vi "Destroy.vi"(8 "error in (no error)":errorcluster, 11 "Array In":refnum<class "Array.lvclass">) -> (0 "error out":errorcluster, 7 "MapImp out":refnum<class "Array.lvclass">)   [LabVIEW 2013, in "LapDog.Collections.v_.Maps.Implementations.lvlib" / "Array.lvclass"]
uses:
  Array.lvclass
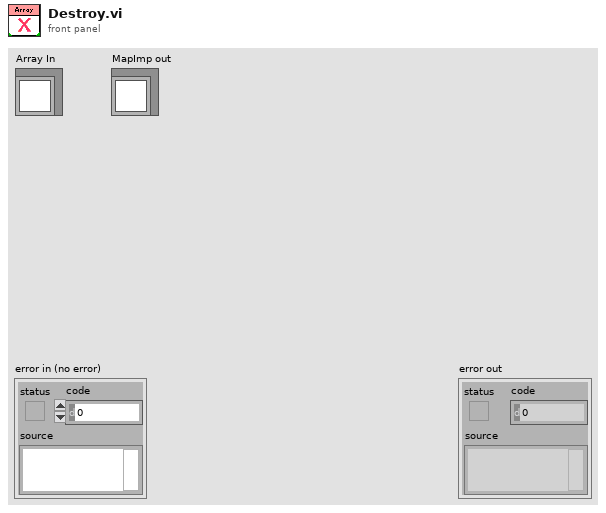
[diagram p1: front panel]
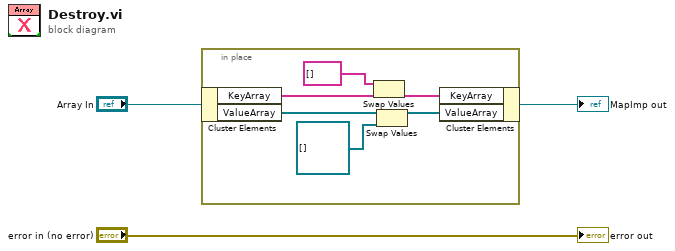
[diagram p0: block diagram]
diagram:
  n1 = in-place {
    n2 = in-place-cluster #1("Array In") -> ("KeyArray"=w7:string[], "ValueArray"=w5:refnum<class>[])
    n3 = Swap Values(12:string[] [] ("KeyArray"), 14:w7) -> (3:w6:string[])  [unwired: 1 in, 1 out]
    n4 = Swap Values(12:w5, 14:refnum<class>[] [] ("ValueArray")) -> (1:w4:refnum<class>[])  [unwired: 1 in, 1 out]
    n5 = in-place-cluster #1("KeyArray"=w6, "ValueArray"=w4) -> (→"MapImp out":refnum<class "Array.lvclass">)
  }
  "error out" <- "error in (no error)"
